vi "Is Theory.vi"(11 "ProjectItem Refnum":refnum<vi>) -> (2 "Is Theory":bool)   [LabVIEW 2017, in "LVUnit Test Discoverer.lvclass"]
uses:
  LVUnit Test Discoverer.lvclass
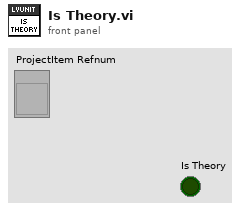
[diagram p1: front panel]
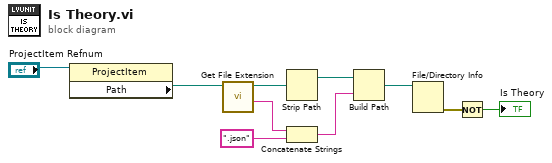
[diagram p0: block diagram]
diagram:
  n1 = property class="ProjectItem"(reference="ProjectItem Refnum") -> ("Path"=w9:path)  [unwired: 1 in, 2 out]
  n2 = call <vilib>:"Get File Extension.vi"("file"=w9) -> ("filename without extension"=w5:string, "dup file"=w8:path)  [unwired: 6 in, 3 out]
  n3 = Strip Path(path=w8) -> (stripped path=w7:path)  [unwired: 1 out]
  n4 = Concatenate Strings(w5, ".json") -> (w4:string)
  n5 = Build Path(base path=w7, name or relative path=w4) -> (appended path=w3:path)
  n6 = File/Directory Info(path=w3) -> (error out=w2:errorcluster)  [unwired: 1 in, 6 out]
  n7 = Not(x=w2) -> (.not. x?=→"Is Theory":bool)
